vi "BIO_pop.vi"(8 "error in (no error)":errorcluster, 11 "BIO in":refnum<class "BIO.lvclass">) -> (0 "error out":errorcluster, 2 "Popped BIO":refnum<class "BIO.lvclass">, 3 "BIO out":refnum<class "BIO.lvclass">)   [LabVIEW 2013, in "OpenSSL Socket.lvlib" / "BIO.lvclass"]
uses:
  BIO.lvclass
  SSL-Lib/SSL-Lib.lvclass/SSL-Lib.ctl
  BIO.lvclass/BIO.ctl
  SSL-Lib/Read Crypto Library Path.vi
  Read Handle.vi
  Write Handle.vi
  SSL-Lib/SSL-Lib.lvclass
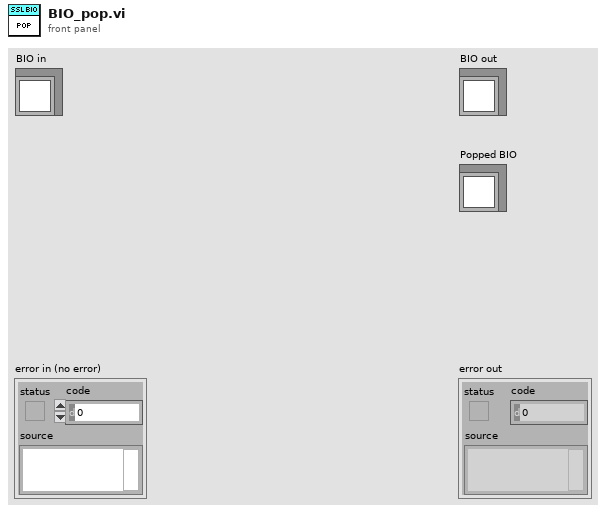
[diagram p1: front panel]
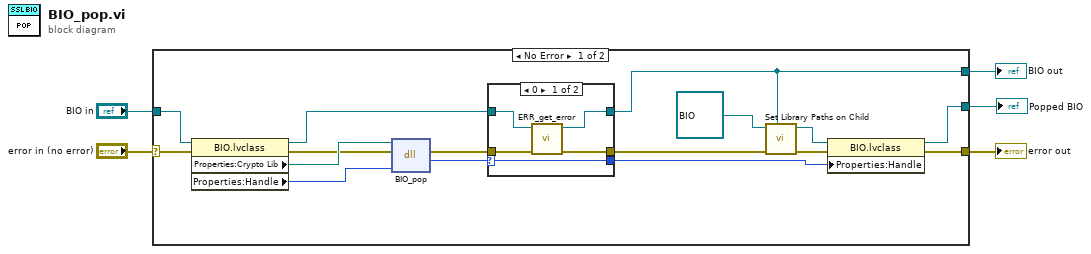
[diagram p0: block diagram]
diagram:
  n1 = case shown="No Error" "error in (no error)" {
    selector: "error in (no error)" -> [w20 w31]
    tunnel: [w9 w31] -> w4
    tunnel: [w11 w30] -> w2
    tunnel: "BIO in" -> [w21 w30]
    tunnel: [w8 _] -> w1
    frame No Error {
      n2 = property class="BIO.lvclass"(reference=w21, error in=w20) -> (reference out=w14:refnum<class "BIO.lvclass">, error out=w17:errorcluster, "Properties:Crypto Lib"=w19:path, "Properties:Handle"=w18:u64)
      n3 = dll-call lib="C:/Program Files (x86)/National Instruments/Shared/nissl/NIlibeay32.dll" fn="BIO_pop"(path in=w19, error in=w17, "BIO"=w18) -> (error out=w15:errorcluster, "return type"=w16:u64)  [unwired: 2 in, 1 out]
      n4 = case shown="0" w16 {
        selector: w16 -> [w22 w27]
        tunnel: w15 -> [w26 w29]
        tunnel: [w23 w29] -> w13
        tunnel: w14 -> [w25 w28]
        tunnel: [w24 w28] -> w11
        tunnel: [w22 w27] -> w6
        frame 0 {
          n5 = call "ERR_get_error.vi"("error in (no error)"=w26, "SSL-Lib in"=w25) -> ("error out"=w23:errorcluster, "SSL-Lib out"=w24:refnum<class "BIO.lvclass">)  [unwired: 8 in]
        }
        frame Default {
        }
      }
      n6 = call-dynamic "Set Library Paths on Child.vi"(7:"SSL-Lib in"=w11, "error in (no error)"=w13, 11:"SSL-Lib in"=refnum<class "BIO.lvclass"> refnum ("Popped BIO")) -> ("error out"=w12:errorcluster, "SSL-Lib out"=w10:refnum<class "BIO.lvclass">)  [unwired: 7 in]
      n7 = property class="BIO.lvclass"(reference=w10, error in=w12, "Properties:Handle"=w6) -> (reference out=w8:refnum<class "BIO.lvclass">, error out=w9:errorcluster)
    }
    frame Error {
    }
  }
  "error out" <- w4
  "BIO out" <- w2
  "Popped BIO" <- w1
